vi "ArdnoLED.vi"() -> ()   [LabVIEW 2018, in "Arduino.lvlib"]
uses:
  Backup LabVIEW Arduino Connection/LINX/Public/Peripherals/Digital/Digital Write 1 Chan.vi
  Arduino.lvlib
  Backup LabVIEW Arduino Connection/LINX/LVH-LINX.lvlib
panel:
  in  "stop":bool
  out "Boolean 2":bool
  in  "Boolean":bool
  out "error out 2":errorcluster
  out "Device Name":string
  in  "error in (no error)":errorcluster
  in  "VISA resource name":refnum<visa-resource-name>
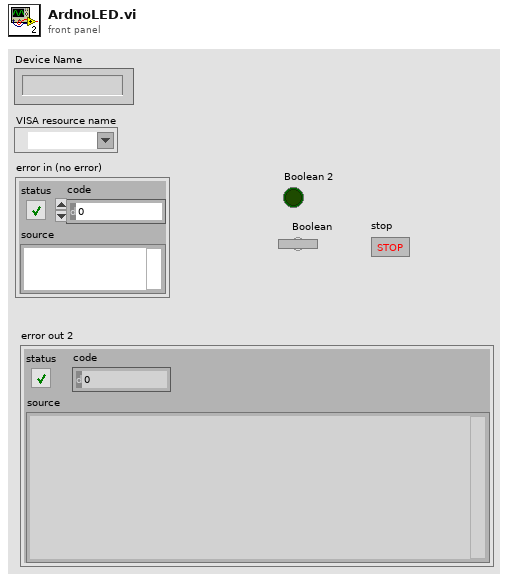
[diagram p1: front panel]
types:
  T1 = typedef "LVH-LINX.lvlib/LINX Ref.ctl" = cluster{"Platform":T2, "Interface":T3, "LINX Device Config":T4}
  T2 = typedef "LVH-LINX.lvlib/Platform.ctl" = enum16{"LINX", "myRIO"}
  T3 = typedef "LVH-LINX.lvlib/Interface.ctl" = enum16{"Serial", "TCP"}
  T4 = typedef "LVH-LINX.lvlib/Device.lvlib/LINX Device Config.ctl" = cluster{"Interface":T3, "COM Port":refnum<visa-resource-name>, "TCP Configuration":T5, "Device Family":T6, "Device ID":u8, "Device Name":string, "TCP Ref":refnum<k5>}
  T5 = typedef "LVH-LINX.lvlib/Device.lvlib/TCP Config.ctl" = cluster{"IP Address":string, "Port":u16}
  T6 = typedef "LVH-LINX.lvlib/Device Family.ctl" = enum8{"National Instruments", "Digilent", "Arduino"}
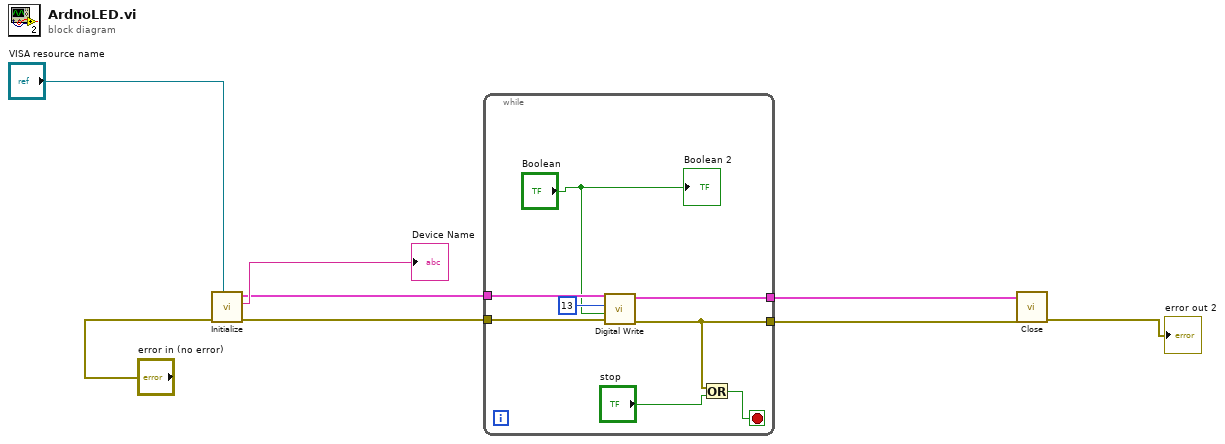
[diagram p0: block diagram]
diagram:
  n1 = call "Initialize.vi"("Serial Port"="VISA resource name", "Error In"="error in (no error)") -> ("Error Out"=w2:errorcluster, "Device Name"=→"Device Name":string, "LINX Ref"=w4:T1)  [unwired: 7 in]
  n2 = while {
    tunnel: w4 -> [w16]
    tunnel: [w15] -> w3
    tunnel: w2 -> [w14]
    tunnel: [w9] -> w1
    stop <- w10 stop-if-true
    n3 = call-poly "Digital Write.vi"("Error In"=w14, "Output Value"="Boolean", "DO Channel"=u8 13, "LINX Resource"=w16) -> ("Error Out"=w9:errorcluster, "LINX Resource"=w15:T1)  [unwired: 6 in]
    n4 = Or(x=w9, y="stop") -> (x .or. y?=w10:bool)
    "Boolean 2" <- "Boolean"
  }
  n5 = call "Close.vi"("Error In"=w1, "LINX Resource"=w3) -> ("Error Out"=→"error out 2":errorcluster)  [unwired: 8 in, 1 out]
